vi "ReportLocalPoseDecode.vi"(1 "Payload":string) -> (0 "LocalPose":T1)   [LabVIEW 2009]
uses:
  Support Files/LocalPose.ctl
  Support Files/TimeRec.ctl
panel:
  out "Presence Vector":u16 format="%b"
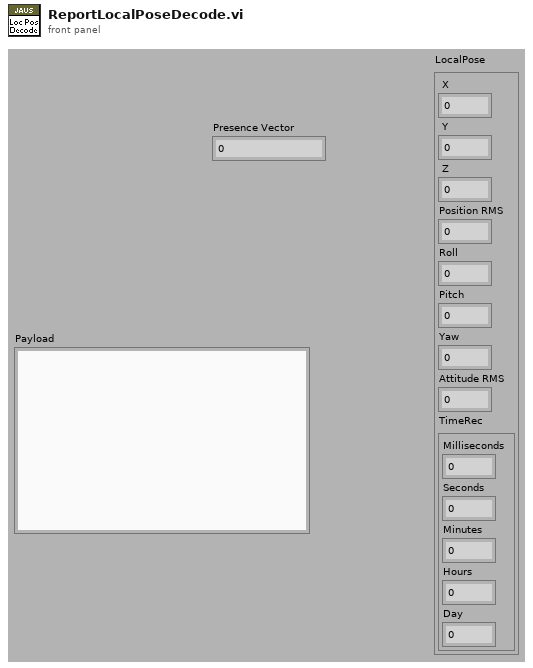
[diagram p1: front panel]
types:
  T1 = typedef "LocalPose.ctl" = cluster{" X":dbl, " Y":dbl, " Z":dbl, "Position RMS":dbl, "Roll":dbl, "Pitch":dbl, "Yaw":dbl, "Attitude RMS":dbl, "TimeRec":T2}
  T2 = typedef "TimeRec.ctl" = cluster{"Milliseconds":u32, "Seconds":u32, "Minutes":u32, "Hours":u32, "Day":u32}
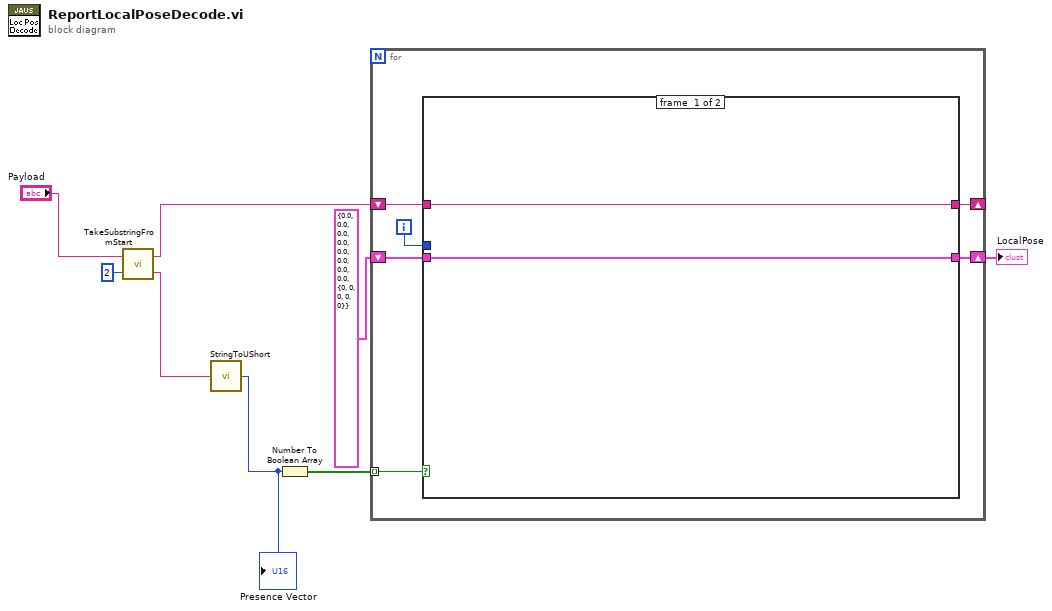
[diagram p0: block diagram]
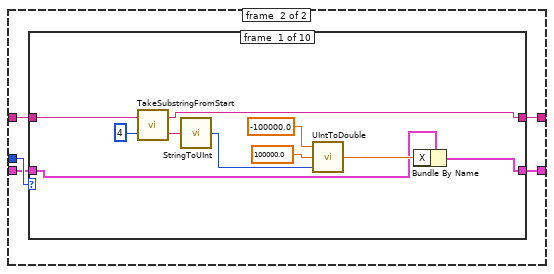
[diagram p2: hidden frame]
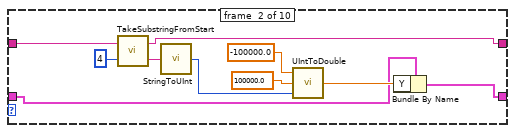
[diagram p3: hidden frame]
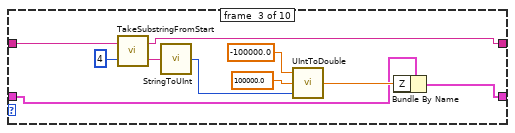
[diagram p4: hidden frame]
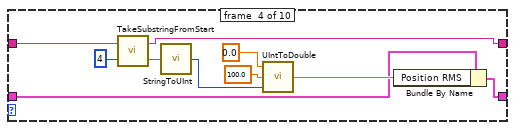
[diagram p5: hidden frame]
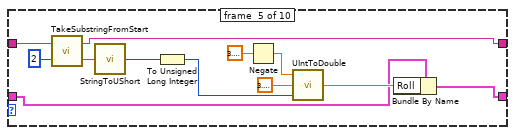
[diagram p6: hidden frame]
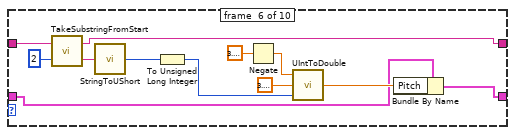
[diagram p7: hidden frame]
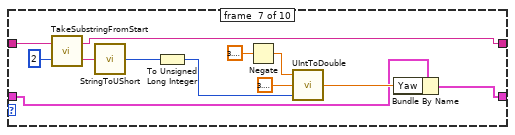
[diagram p8: hidden frame]
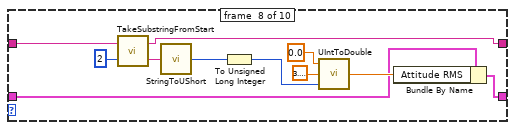
[diagram p9: hidden frame]
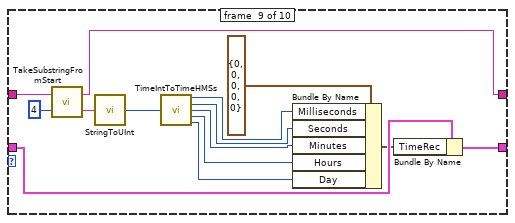
[diagram p10: hidden frame]
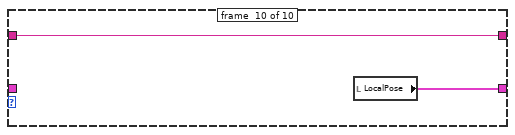
[diagram p11: hidden frame]
diagram:
  n1 = call "TakeSubstringFromStart.vi"("offset"=2, "string"="Payload") -> ("string before offset"=w4:string, "string after offset"=w2:string)
  n2 = call "StringToUShort.vi"("string"=w4) -> ("UShort"=w3:u16)
  "Presence Vector" <- w3
  n3 = Number To Boolean Array(number=w3) -> (Boolean array=w1:bool[])
  n4 = for {
    tunnel: w1 -> [w13] mode=indexing
    shift-right: [w11] -> w7
    shift-left: T1 {" X"=0.0, " Y"=0.0, " Z"=0.0, "Position RMS"=0.0, "Roll"=0.0, "Pitch"=0.0, "Yaw"=0.0, "Attitude RMS"=0.0, "TimeRec"={"Milliseconds"=0, "Seconds"=0, "Minutes"=0, "Hours"=0, "Day"=0}} ("LocalPose") -> [w12]
    shift-right: [w10] -> _
    shift-left: w2 -> [w9]
    i -> [w14]
    n5 = case shown="True" w13 {
      tunnel: w14 -> [_ w21]
      tunnel: w9 -> [w15 w20]
      tunnel: w12 -> [w16 w19]
      tunnel: [w16 w18] -> w11
      tunnel: [w15 w17] -> w10
      frame #0 {
      }
      frame #1 {
        n6 = case shown="1" w21 {
          tunnel: w20 -> [w30 w40 w50 w60 w72 w84 w96 w107 w121 w123]
          tunnel: w19 -> [w25 w35 w45 w54 w65 w77 w88 w100 w114 _]
          tunnel: [w24 w34 w44 w55 w66 w76 w89 w101 w112 w124] -> w18
          tunnel: [w22 w33 w42 w52 w64 w74 w87 w99 w109 w123] -> w17
          frame #0 {
            n7 = call "TakeSubstringFromStart.vi"("offset"=4 ("reduce by"), "string"=w30) -> ("string before offset"=w23:string, "string after offset"=w22:string)
            n8 = call "StringToUInt.vi"("string"=w23) -> ("UInt"=w29:u32)
            n9 = call "UIntToDouble.vi"("Value"=w29, "Max"=100000.0, "Min"=-100000.0) -> ("Number"=w26:dbl)
            n10 = Bundle By Name(cluster=w25, "X"=w26) -> (w24:T1)
          }
          frame #1 {
            n11 = call "TakeSubstringFromStart.vi"("offset"=4 ("reduce by"), "string"=w40) -> ("string before offset"=w32:string, "string after offset"=w33:string)
            n12 = call "StringToUInt.vi"("string"=w32) -> ("UInt"=w39:u32)
            n13 = call "UIntToDouble.vi"("Value"=w39, "Max"=100000.0, "Min"=-100000.0) -> ("Number"=w36:dbl)
            n14 = Bundle By Name(cluster=w35, "Y"=w36) -> (w34:T1)
          }
          frame #2 {
            n15 = call "TakeSubstringFromStart.vi"("offset"=4 ("reduce by"), "string"=w50) -> ("string before offset"=w43:string, "string after offset"=w42:string)
            n16 = call "StringToUInt.vi"("string"=w43) -> ("UInt"=w49:u32)
            n17 = call "UIntToDouble.vi"("Value"=w49, "Max"=100000.0, "Min"=-100000.0) -> ("Number"=w46:dbl)
            n18 = Bundle By Name(cluster=w45, "Z"=w46) -> (w44:T1)
          }
          frame #3 {
            n19 = call "TakeSubstringFromStart.vi"("offset"=4 ("reduce by"), "string"=w60) -> ("string before offset"=w53:string, "string after offset"=w52:string)
            n20 = call "StringToUInt.vi"("string"=w53) -> ("UInt"=w59:u32)
            n21 = call "UIntToDouble.vi"("Value"=w59, "Max"=100.0, "Min"=0.0) -> ("Number"=w56:dbl)
            n22 = Bundle By Name(cluster=w54, "Position RMS"=w56) -> (w55:T1)
          }
          frame #4 {
            n23 = call "TakeSubstringFromStart.vi"("offset"=2 ("reduce by"), "string"=w72) -> ("string before offset"=w62:string, "string after offset"=w64:string)
            n24 = call "StringToUShort.vi"("string"=w62) -> ("UShort"=w63:u16)
            n25 = To Unsigned Long Integer(number=w63) -> (unsigned 32bit integer=w68:u32)
            n26 = Negate(x=3.141592653589793) -> (-x=w70:dbl)
            n27 = call "UIntToDouble.vi"("Value"=w68, "Max"=3.141592653589793, "Min"=w70) -> ("Number"=w67:dbl)
            n28 = Bundle By Name(cluster=w65, "Roll"=w67) -> (w66:T1)
          }
          frame #5 {
            n29 = call "TakeSubstringFromStart.vi"("offset"=2 ("reduce by"), "string"=w84) -> ("string before offset"=w75:string, "string after offset"=w74:string)
            n30 = call "StringToUShort.vi"("string"=w75) -> ("UShort"=w83:u16)
            n31 = To Unsigned Long Integer(number=w83) -> (unsigned 32bit integer=w79:u32)
            n32 = Negate(x=3.141592653589793) -> (-x=w81:dbl)
            n33 = call "UIntToDouble.vi"("Value"=w79, "Max"=3.141592653589793, "Min"=w81) -> ("Number"=w78:dbl)
            n34 = Bundle By Name(cluster=w77, "Pitch"=w78) -> (w76:T1)
          }
          frame #6 {
            n35 = call "TakeSubstringFromStart.vi"("offset"=2 ("reduce by"), "string"=w96) -> ("string before offset"=w86:string, "string after offset"=w87:string)
            n36 = call "StringToUShort.vi"("string"=w86) -> ("UShort"=w95:u16)
            n37 = To Unsigned Long Integer(number=w95) -> (unsigned 32bit integer=w91:u32)
            n38 = Negate(x=3.141592653589793) -> (-x=w93:dbl)
            n39 = call "UIntToDouble.vi"("Value"=w91, "Max"=3.141592653589793, "Min"=w93) -> ("Number"=w90:dbl)
            n40 = Bundle By Name(cluster=w88, "Yaw"=w90) -> (w89:T1)
          }
          frame #7 {
            n41 = call "TakeSubstringFromStart.vi"("offset"=2 ("reduce by"), "string"=w107) -> ("string before offset"=w98:string, "string after offset"=w99:string)
            n42 = call "StringToUShort.vi"("string"=w98) -> ("UShort"=w106:u16)
            n43 = To Unsigned Long Integer(number=w106) -> (unsigned 32bit integer=w104:u32)
            n44 = call "UIntToDouble.vi"("Value"=w104, "Max"=3.141592653589793, "Min"=0.0) -> ("Number"=w102:dbl)
            n45 = Bundle By Name(cluster=w100, "Attitude RMS"=w102) -> (w101:T1)
          }
          frame #8 {
            n46 = call "TakeSubstringFromStart.vi"("offset"=4 ("reduce by"), "string"=w121) -> ("string before offset"=w110:string, "string after offset"=w109:string)
            n47 = call "StringToUInt.vi"("string"=w110) -> ("UInt"=w111:u32)
            n48 = call "TimeIntToTimeHMSs.vi"("Time Int"=w111) -> ("Milliseconds"=w119:u32, "Seconds"=w118:u32, "Minutes"=w117:u32, "Hours"=w116:u32, "Day"=w115:u32)  [unwired: 10 in]
            n49 = Bundle By Name(cluster=T2 {"Milliseconds"=0, "Seconds"=0, "Minutes"=0, "Hours"=0, "Day"=0} ("TimeRec"), "Milliseconds"=w119, "Seconds"=w118, "Minutes"=w117, "Hours"=w116, "Day"=w115) -> (w113:T2)
            n50 = Bundle By Name(cluster=w114, "TimeRec"=w113) -> (w112:T1)
          }
          frame #9 {
            n51 = local read "LocalPose"() -> (w124:T1)
          }
        }
      }
    }
  }
  "LocalPose" <- w7
